vi "exists.vi"(8 "error in (no error)":errorcluster, 10 "Key":string, 11 "Bucket in":refnum<class "Bucket.lvclass">) -> (0 "error out":errorcluster, 2 "Exists?":bool, 3 "Bucket out":refnum<class "Bucket.lvclass">)   [LabVIEW 2017, in "Bucket.lvclass"]
uses:
  <userlib>/836-Library/Data_Structures/Bucket/Bucket.lvclass
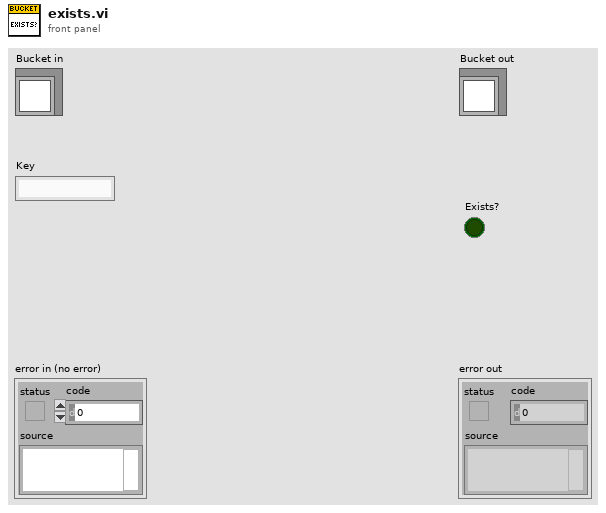
[diagram p1: front panel]
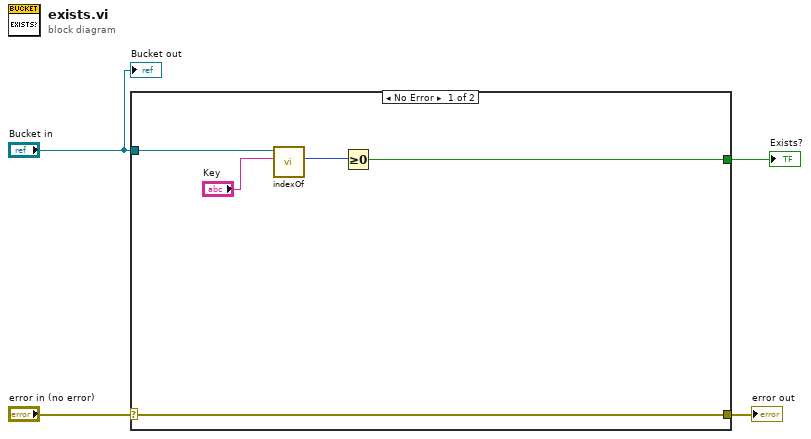
[diagram p0: block diagram]
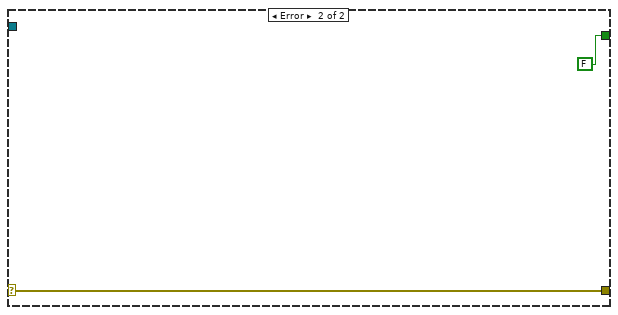
[diagram p2: hidden frame]
diagram:
  n1 = case shown="No Error" "error in (no error)" {
    selector: "error in (no error)" -> [w9 w11]
    tunnel: [w9 w11] -> w3
    tunnel: "Bucket in" -> [w8 _]
    tunnel: [w5 FALSE] -> w1
    frame No Error {
      n2 = call <userlib>:"indexOf.vi"("Key"="Key", "Bucket in"=w8) -> ("Index"=w6:i32)  [unwired: 7 in, 2 out]
      n3 = Greater Or Equal To 0?(x=w6) -> (x >= 0?=w5:bool)
    }
    frame Error {
    }
  }
  "error out" <- w3
  "Exists?" <- w1
  "Bucket out" <- "Bucket in"
